vi "API example.vi"() -> ()   [LabVIEW 2013]
uses:
  collection/VI modification collection.lvclass
  tools/set source separate/set source separate.lvclass
  tools/set source separate/set source separate.lvclass/set source separate.ctl
  tools/set source separate/Write separate compiled code.vi
panel:
  in  "Path":path
  out "error report":errorcluster[](array[cluster])
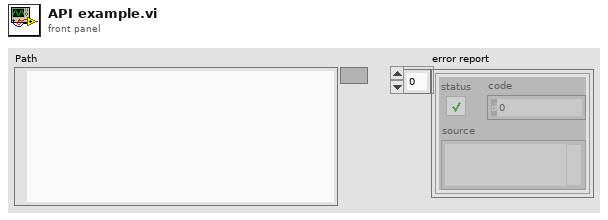
[diagram p1: front panel]
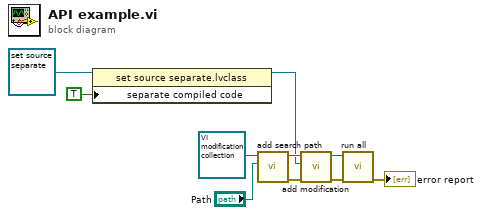
[diagram p0: block diagram]
diagram:
  n1 = property class="set source separate.lvclass"(reference=refnum<class "set source separate.lvclass"> refnum ("set source separate.lvclass"), "separate compiled code"=TRUE) -> (reference out=w1:refnum<class "set source separate.lvclass">)  [unwired: 1 in, 1 out]
  n2 = call "add search path.vi"("Path"="Path", "vi modification tool in"=refnum<class "VI modification collection.lvclass"> refnum ("vi modification tool.lvclass")) -> ("error out"=w5:errorcluster, "vi modification tool out"=w4:refnum<class "VI modification collection.lvclass">)  [unwired: 8 in]
  n3 = call "add modification.vi"("error in"=w5, "VI modification"=w1, "vi modification tool in"=w4) -> ("error out"=w2:errorcluster, "vi modification tool out"=w3:refnum<class "VI modification collection.lvclass">)  [unwired: 7 in]
  n4 = call "run all.vi"("error in"=w2, "vi modification tool in"=w3) -> ("error report"=→"error report":errorcluster[])  [unwired: 8 in, 1 out]
